vi "22_DC Motor_PID_final_deploy.vi"() -> ()   [LabVIEW 2018]
uses:
  <userlib>/KNR OS 4.0 LabVIEW Toolkit/Type Definition/Resource.ctl
  <userlib>/KNR OS 4.0 LabVIEW Toolkit/Type Definition/DC Motor Port.ctl
panel:
  in  "Reset 2":bool
  in  "Reverse? 2":bool
  out "Velocity (cm/sec) 2":dbl
  out "Position cm 2":dbl
  out "Speed (+-100%) 2":dbl
  out "Speed (+-100%)":dbl
  in  "IP":string(combo)="172.22.11.2"
  in  "Resource":T1=enum."KNRm_DDDD"
  in  "stop":bool
  out "Position cm":dbl
  out "Velocity (cm/sec)":dbl
  in  "Reverse?":bool
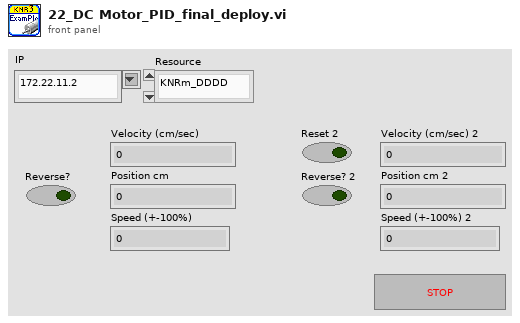
[diagram p1: front panel]
types:
  T1 = typedef "Resource.ctl" = enum16{"KNRm_DDRC", "KNRm_DDDD", "KNRm_DDDR", "KNRm_DDDC", "KNR", "KNRm_neww"}
  T2 = typedef "KNR3 Reference.ctl" = cluster{"FPGA Session":refnum<class "FPGA Interface Base.lvclass">, "Resource":T1}
  T3 = typedef "DC Motor Port.ctl" = u16
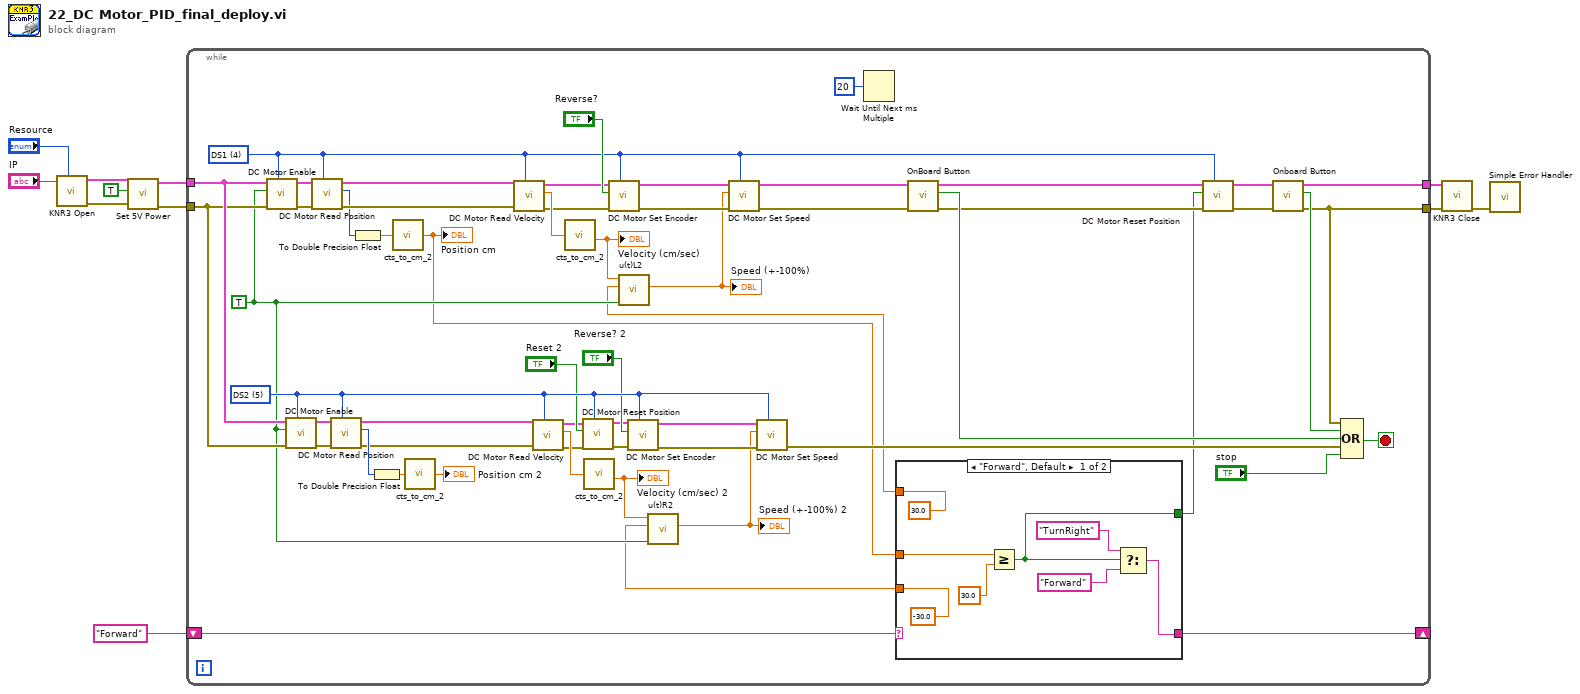
[diagram p0: block diagram]
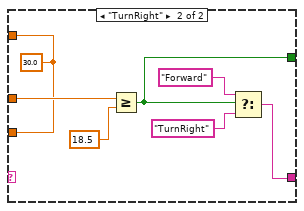
[diagram p2: hidden frame]
diagram:
  n1 = call <userlib>:"KNR3 Open.vi"("Resource"="Resource", "IP"="IP") -> ("error out"=w5:errorcluster, "KNR out"=w7:T2)  [unwired: 8 in]
  n2 = call <userlib>:"Set 5V Power.vi"("error in (no error)"=w5, "5V Power(T)"=TRUE ("5V Power"), "KNR in"=w7) -> ("error out"=w9:errorcluster, "KNR out"=w10:T2)  [unwired: 7 in]
  n3 = while {
    tunnel: w10 -> [w33]
    tunnel: w9 -> [w32]
    tunnel: [w14] -> w3
    tunnel: [w12] -> w2
    shift-right: [w16] -> _
    shift-left: "Forward" -> [w26]
    stop <- w66 stop-if-true
    w29 = TRUE ("Enable Motor")
    w50 = T3 5 items=["DS1"=4, "DS2"=5, "DS3"=6, "DS4"=7] ("Port 2")
    w54 = T3 4 items=["DS1"=4, "DS2"=5, "DS3"=6, "DS4"=7] ("Port")
    n4 = call <userlib>:"DC Motor Enable.vi"("Port (DS1)"=w54, "error in (no error)"=w32, "Enable Motor(F)"=w29, "KNR in"=w33) -> ("error out"=w57:errorcluster, "KNR out"=w58:T2)  [unwired: 6 in]
    n5 = call <userlib>:"DC Motor Enable.vi"("Port (DS1)"=w50, "error in (no error)"=w32, "Enable Motor(F)"=w29, "KNR in"=w33) -> ("error out"=w47:errorcluster, "KNR out"=w46:T2)  [unwired: 6 in]
    n6 = call <userlib>:"DC Motor Read Position.vi"("Port (DS1)"=w54, "error in (no error)"=w57, "KNR in"=w58) -> ("error out"=w63:errorcluster, "Position"=w60:i32, "KNR out"=w64:T2)  [unwired: 6 in]
    n7 = call <userlib>:"DC Motor Read Position.vi"("Port (DS1)"=w50, "error in (no error)"=w47, "KNR in"=w46) -> ("error out"=w35:errorcluster, "Position"=w44:i32, "KNR out"=w34:T2)  [unwired: 6 in]
    n8 = To Double Precision Float(number=w60) -> (double precision float=w59:dbl)
    n9 = To Double Precision Float(number=w44) -> (double precision float=w45:dbl)
    n10 = call "cts_to_cm_2.vi"("cts"=w59) -> ("cm"=w24:dbl)
    "Position cm" <- w24
    n11 = call "cts_to_cm_2.vi"("cts"=w45) -> ("cm"=→"Position cm 2":dbl)
    n12 = call <userlib>:"DC Motor Read Velocity.vi"("Port (DS1)"=w54, "error in (no error)"=w63, "KNR in"=w64) -> ("error out"=w20:errorcluster, "Velocity (cts/sec)"=w62:dbl, "KNR out"=w21:T2)  [unwired: 6 in]
    n13 = call <userlib>:"DC Motor Read Velocity.vi"("Port (DS1)"=w50, "error in (no error)"=w35, "KNR in"=w34) -> ("error out"=w39:errorcluster, "Velocity (cts/sec)"=w40:dbl, "KNR out"=w36:T2)  [unwired: 6 in]
    n14 = call "cts_to_cm_2.vi"("cts"=w62) -> ("cm"=w52:dbl)
    "Velocity (cm/sec)" <- w52
    n15 = call <userlib>:"DC Motor Reset Position.vi"("Port (DS1)"=w50, "error in (no error)"=w39, "Reset(F)"="Reset 2", "KNR in"=w36) -> ("error out"=w38:errorcluster, "KNR out"=w37:T2)  [unwired: 6 in]
    n16 = call "cts_to_cm_2.vi"("cts"=w40) -> ("cm"=w30:dbl)
    "Velocity (cm/sec) 2" <- w30
    n17 = call <userlib>:"DC Motor Set Encoder.vi"("Port (DS1)"=w54, "error in (no error)"=w20, "Reverse?(F)"="Reverse?", "KNR in"=w21) -> ("error out"=w55:errorcluster, "KNR out"=w56:T2)  [unwired: 6 in]
    n18 = call <userlib>:"DC Motor Set Encoder.vi"("Port (DS1)"=w50, "error in (no error)"=w38, "Reverse?(F)"="Reverse? 2", "KNR in"=w37) -> ("error out"=w49:errorcluster, "KNR out"=w48:T2)  [unwired: 6 in]
    n19 = Wait Until Next ms Multiple(millisecond multiple=u32 20) -> ()  [unwired: 1 out]
    n20 = case shown="\"Forward\", Default" w26 {
      tunnel: [30.0 w78] -> w25
      tunnel: w24 -> [w71 w79]
      tunnel: [-30.0 w78] -> w23
      tunnel: [w69 w76] -> w16
      tunnel: [w68 w77] -> w15
      frame "Forward", Default {
        n21 = Greater Or Equal?(x=w71, y=30.0) -> (x >= y?=w68:bool)
        n22 = Select(t="TurnRight", s=w68, f="Forward") -> (s? t:f=w69:string)
      }
      frame "TurnRight" {
        w78 = 30.0
        n23 = Greater Or Equal?(x=w79, y=18.5) -> (x >= y?=w77:bool)
        n24 = Select(t="Forward", s=w77, f="TurnRight") -> (s? t:f=w76:string)
      }
    }
    n25 = call "u(t)L2.vi"("Velocity"=w52, "Desire Velosity"=w25, "enable"=w29) -> ("u(t)"=w51:dbl)  [unwired: 7 in]
    "Speed (+-100%)" <- w51
    n26 = call "u(t)R2.vi"("Velocity"=w30, "Desire Velosity"=w23, "enable"=w29) -> ("u(t)"=w28:dbl)  [unwired: 7 in]
    "Speed (+-100%) 2" <- w28
    n27 = call <userlib>:"DC Motor Set Speed.vi"("Port (DS1)"=w54, "error in (no error)"=w55, "Speed (+-100%)"=w51, "KNR in"=w56) -> ("error out"=w19:errorcluster, "KNR out"=w53:T2)  [unwired: 6 in]
    n28 = call <userlib>:"DC Motor Set Speed.vi"("Port (DS1)"=w50, "error in (no error)"=w49, "Speed (+-100%)"=w28, "KNR in"=w48) -> ("error out"=w31:errorcluster)  [unwired: 6 in, 1 out]
    n29 = call <userlib>:"OnBoard Button.vi"("error in (no error)"=w19, "KNR in"=w53) -> ("error out"=w18:errorcluster, "value"=w27:bool, "KNR out"=w22:T2)  [unwired: 7 in]
    n30 = call <userlib>:"DC Motor Reset Position.vi"("Port (DS1)"=w54, "error in (no error)"=w18, "Reset(F)"=w15, "KNR in"=w22) -> ("error out"=w12:errorcluster, "KNR out"=w17:T2)  [unwired: 6 in]
    n31 = call <userlib>:"Onboard Button.vi"("KNR in"=w17) -> ("value"=w13:bool, "KNR out"=w14:T2)  [unwired: 8 in, 1 out]
    n32 = Compound Arithmetic op=OR(w12, w13, w27, w31, "stop") -> (w66:bool)
  }
  n33 = call <userlib>:"KNR3 Close.vi"("error in (no error)"=w2, "KNR in"=w3) -> ("error out"=w8:errorcluster)  [unwired: 9 in]
  n34 = call <vilib>:"Simple Error Handler.vi"("error in (no error)"=w8) -> ()  [unwired: 4 in, 5 out]
